vi "tb_push and pop with known sequence.vi"(9 "fifo depth":u8(ring)=10 items=["4"=2, "8"=3, "16"=4, "32"=5, "64"=6, "128"=7, "256"=8, "512"=9, "1024"=10, "2048"=11, "4096"=12, "8192"=13, "16384"=14, "32768"=15, "65536"=16, "131072"=17, "262144"=18, "524288"=19, "1048576"=20, "2097152"=21, "4194304"=22, "8388608"=23, "16777216"=24, "33554432"=25, "67108864"=26, "134217728"=27, "268435456"=28, "536870912"=29, "1073741824"=30, "2147483648"=31, "4294967296"=32], 10 "arbiter configuration":T4={"write grant time (clocks)"=100, "read grant time (clocks)"=100}, 11 "Memory":T5={"fifo1 memory"="Bank0", "fifo2 memory"="Bank1"}) -> (3 "Pass?":bool)   [LabVIEW 2011]
uses:
  Data Type (256).ctl
  <instrlib>/RF-RIO/Memory/FPGA/Interface/Timeslot Arbiter Configuration.ctl
  <instrlib>/RF-RIO/Memory/FPGA/Interface/Retrieve Data (128-Bit).ctl
  <instrlib>/RF-RIO/Memory/FPGA/Interface/U128.ctl
  <instrlib>/RF-RIO/Memory/FPGA/Memory.lvlib
panel:
  out "DataValid":bool[](array[boolean])
  out "Bank1.Data":T1[](array[typedef])
  out "Bank0.Data":T1[](array[typedef])
  out "Output Data":T3[](array[typedef])
  out "Iteration":i32
  out "FIFO Input":T3[](array[typedef])
  out "FIFO Output":T3[](array[typedef])
  # "This VI tests the FIFO with known Sequence: Linear Ramp"
  # "Debug Area"
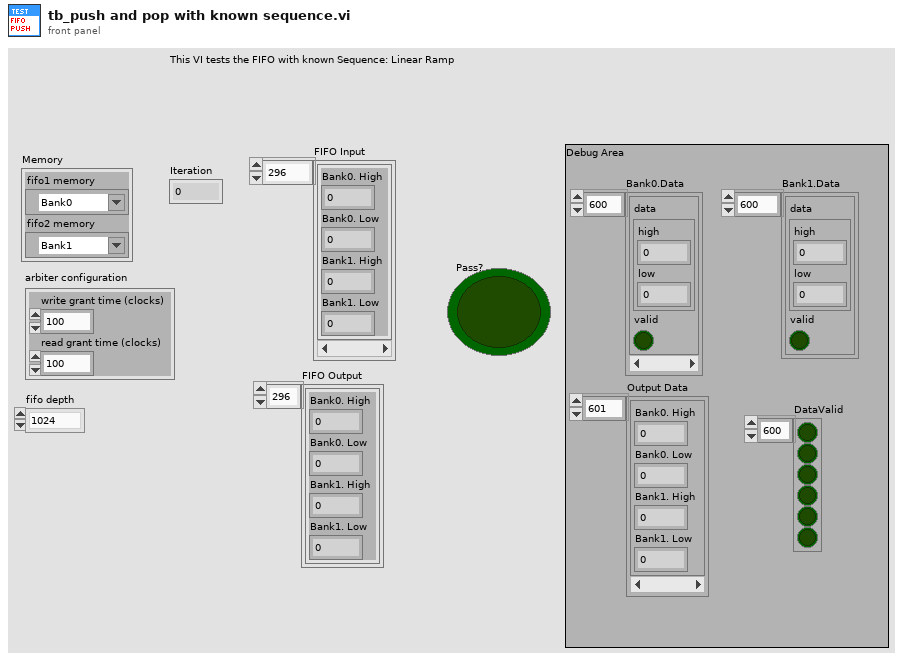
[diagram p1: front panel]
types:
  T1 = typedef "Memory.lvlib/Retrieve Data (128-Bit).ctl" = cluster{"data":T2, "valid":bool}
  T2 = typedef "Memory.lvlib/U128.ctl" = cluster{"high":u64, "low":u64}
  T3 = typedef "Data Type (256).ctl" = cluster{"Bank0. High":u64, "Bank0. Low":u64, "Bank1. High":u64, "Bank1. Low":u64}
  T4 = typedef "Memory.lvlib/Timeslot Arbiter Configuration.ctl" = cluster{"write grant time (clocks)":u16, "read grant time (clocks)":u16}
  T5 = cluster{"fifo1 memory":refnum<k21>, "fifo2 memory":refnum<k21>}
  T6 = cluster{"Bank0. High":bool, "Bank0. Low":bool, "Bank1. High":bool, "Bank1. Low":bool}[]
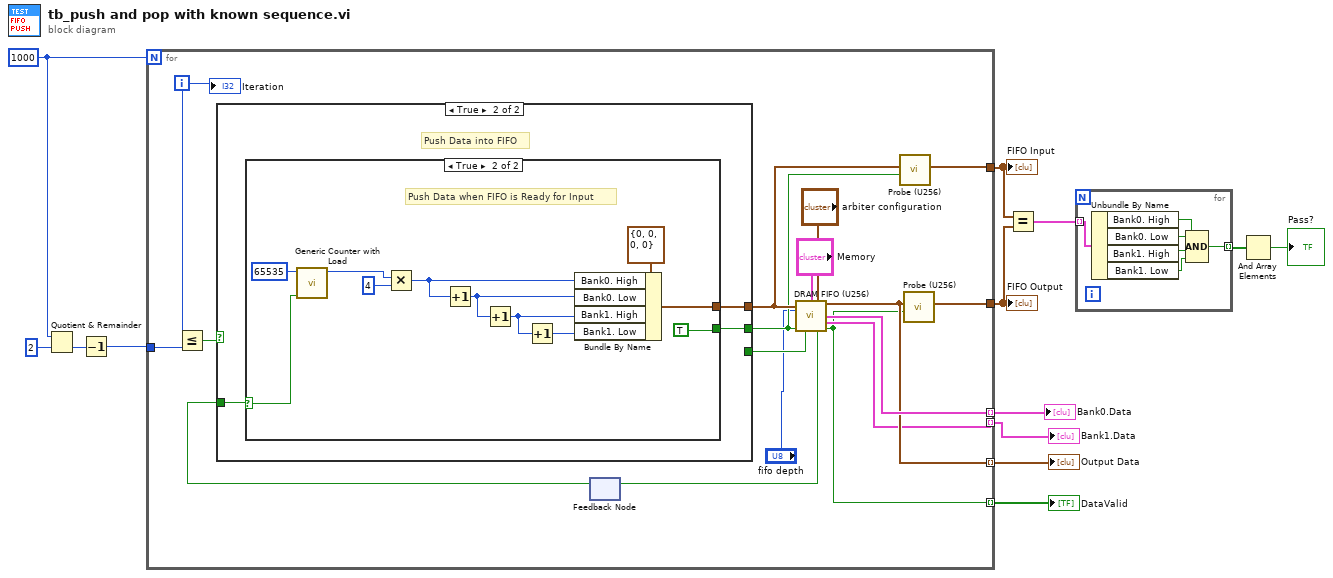
[diagram p0: block diagram]
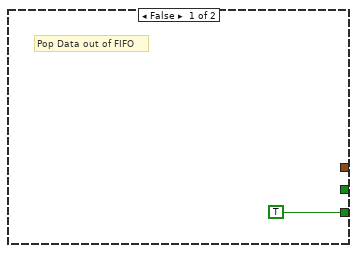
[diagram p2: hidden frame]
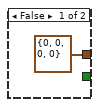
[diagram p3: hidden frame]
diagram:
  w13 = 1000
  n1 = Quotient & Remainder(x=w13, y=2) -> (floor(x/y)=w11:i32)  [unwired: 1 out]
  n2 = Decrement(x=w11) -> (x-1=w10:i32)
  n3 = for {
    N: w13 -> [_]
    tunnel: [w26] -> w8
    tunnel: [w23] -> w9
    tunnel: w10 -> [w20]
    tunnel: [w17] -> w3 mode=indexing
    tunnel: [w16] -> w4 mode=indexing
    tunnel: [w15] -> w2 mode=indexing
    tunnel: [w14] -> w1 mode=indexing
    i -> [w21]
    n4 = Less Or Equal?(x=w21, y=w20) -> (x <= y?=w22:bool)
    n5 = feedback #1() -> (w28:bool)  [unwired: 1 in]
    n6 = case shown="True" w22 {
      tunnel: [_ w34] -> w25
      tunnel: [_ w33] -> w24
      tunnel: w28 -> [_ w32]
      tunnel: [TRUE _] -> w27
      frame False {
        # "Pop Data out of FIFO"
      }
      frame True {
        # "Push Data into FIFO"
        n7 = case shown="True" w32 {
          selector: w32 -> [_ w36]
          tunnel: [T3 {"Bank0. High"=0, "Bank0. Low"=0, "Bank1. High"=0, "Bank1. Low"=0} ("Input Data") w40] -> w34
          tunnel: [_ TRUE] -> w33
          frame False {
          }
          frame True {
            # "Push Data when FIFO is Ready for Input"
            n8 = call "Generic Counter with Load.vi"("INC?"=w36, "rollover"=u16 65535) -> ("count"=w39:u16)  [unwired: 9 in]
            n9 = Multiply(x=w39, y=4) -> (x*y=w44:i32)
            n10 = Increment(x=w44) -> (x+1=w43:i32)
            n11 = Increment(x=w43) -> (x+1=w41:i32)
            n12 = Increment(x=w41) -> (x+1=w42:i32)
            n13 = Bundle By Name(cluster=T3 {"Bank0. High"=0, "Bank0. Low"=0, "Bank1. High"=0, "Bank1. Low"=0} ("Input Data"), "Bank0. High"=w44, "Bank0. Low"=w43, "Bank1. High"=w41, "Bank1. Low"=w42) -> (w40:T3)
          }
        }
      }
    }
    n14 = call "DRAM FIFO (U256).vi"("Input Data"=w25, "Memory"="Memory", "arbiter configuration"="arbiter configuration", "fifo depth"="fifo depth", "input valid"=w24, "ready for output"=w27) -> ("Output Data"=w16:T3, "bank0.data"=w17:T1, "Bank1.data"=w15:T1, "Ready for Input"=w29:bool, "Output Valid"=w14:bool)  [unwired: 5 in]
    n15 = feedback-in #1(w29) -> ()
    n16 = call "Probe (U256).vi"("Data Valid"=w24, "Input"=w25) -> ("Collected Data"=w23:T3[])  [unwired: 8 in, 1 out]
    n17 = call "Probe (U256).vi"("Data Valid"=w14, "Input"=w16) -> ("Collected Data"=w26:T3[])  [unwired: 8 in, 1 out]
    "Iteration" <- w21
  }
  "FIFO Output" <- w8
  "FIFO Input" <- w9
  "Output Data" <- w4
  "Bank0.Data" <- w3
  "Bank1.Data" <- w2
  "DataValid" <- w1
  n18 = Equal?(x=w9, y=w8) -> (x = y?=w7:T6)
  n19 = for {
    tunnel: w7 -> [w52] mode=indexing
    tunnel: [w47] -> w6 mode=indexing
    n20 = Unbundle By Name(w52) -> ("Bank0. High"=w51:bool, "Bank0. Low"=w50:bool, "Bank1. High"=w49:bool, "Bank1. Low"=w48:bool)
    n21 = Compound Arithmetic op=AND(w51, w50, w49, w48) -> (w47:bool)
  }
  n22 = And Array Elements(Boolean array=w6) -> (logical AND=→"Pass?":bool)
